vi "Define Config.vi"(8 "Error In":errorcluster, 9 "Config":refnum<class "IConfig.lvclass">, 10 "Name":string, 11 "Logger In":refnum<class "Logger.lvclass">) -> (0 "Error Out":errorcluster, 3 "Logger Out":refnum<class "Logger.lvclass">)   [LabVIEW 2019, in "Logger.lvclass"]
uses:
  Logger.lvclass
  IConfig/IConfig.lvclass
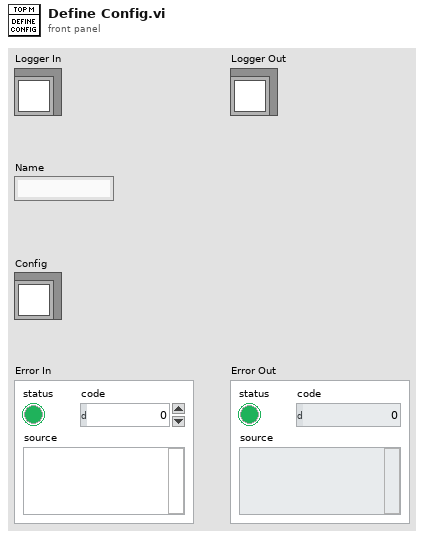
[diagram p1: front panel]
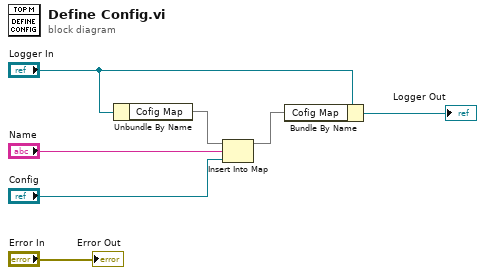
[diagram p0: block diagram]
diagram:
  n1 = Unbundle By Name("Logger In") -> ("Cofig Map"=w5:map{string, refnum<class "IConfig.lvclass">})
  n2 = Insert Into Map(map in=w5, key="Name", value="Config") -> (map out=w6:map{string, refnum<class "IConfig.lvclass">})  [unwired: 2 out]
  n3 = Bundle By Name(cluster="Logger In", "Cofig Map"=w6) -> (→"Logger Out":refnum<class "Logger.lvclass">)
  "Error Out" <- "Error In"
